vi "Read Plugin Options.vi"(8 "error in (no error)":errorcluster, 11 "MeasurementMetaData in":refnum<class "MeasurementMetaData.lvclass">) -> (0 "error out":errorcluster, 2 "Plugin Options":T1, 3 "MeasurementMetaData out":refnum<class "MeasurementMetaData.lvclass">)   [LabVIEW 2013, in "MeasurementMetaData.lvclass"]
uses:
  MeasurementMetaData.lvclass
  Plugin Settings.ctl
  MeasurementMetaData.lvclass/MeasurementMetaData.ctl
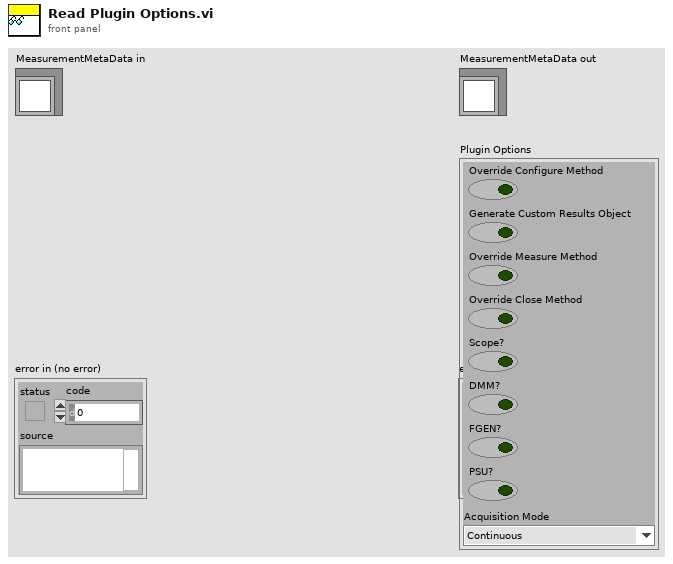
[diagram p1: front panel]
types:
  T1 = typedef "MeasurementMetaData.lvclass/Plugin Settings.ctl" = cluster{"Override Configure Method":bool, "Generate Custom Results Object":bool, "Override Measure Method":bool, "Override Close Method":bool, "Scope?":bool, "DMM?":bool, "FGEN?":bool, "PSU?":bool, "Acquisition Mode":enum16{"Continuous", "Single-Shot"}}
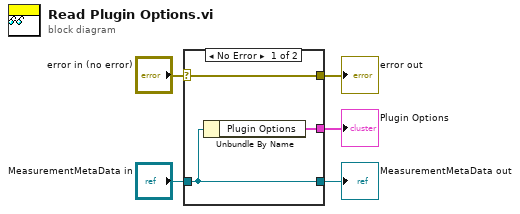
[diagram p0: block diagram]
diagram:
  n1 = case shown="No Error" "error in (no error)" {
    selector: "error in (no error)" -> [w8 w9]
    tunnel: [w8 w9] -> w4
    tunnel: [w7 w10] -> w2
    tunnel: "MeasurementMetaData in" -> [w7 w10]
    tunnel: [w6 _] -> w1
    frame No Error {
      n2 = Unbundle By Name(w7) -> ("Plugin Options"=w6:T1)
    }
    frame Error {
    }
  }
  "error out" <- w4
  "MeasurementMetaData out" <- w2
  "Plugin Options" <- w1
